vi "Revision Query.vi"(8 "error in (no error)":errorcluster, 11 "VISA resource name":refnum<visa-resource-name>) -> (0 "error out":errorcluster, 1 "Instrument Firmware Revision":string, 2 "Instrument Driver Revision":string, 3 "VISA resource name out":refnum<visa-resource-name>)   [LabVIEW 2015, in "Newport ESP301.lvlib"]
doc: "This command is used to read the controller type and version.\n\n<B>NOTE:</B> Important information needed when asking for technical support for the motion control system or when reporting a problem is the controller version. Use this command to determine the controller type and in particular, the firmware version.\n\nRefer to the Readme file for detailed driver information including modification history."
uses:
  <userlib>/Newport ESP301/Newport ESP301.lvlib
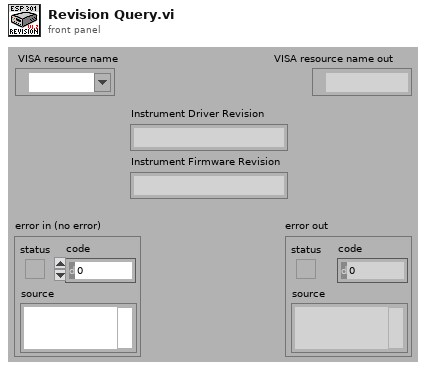
[diagram p1: front panel]
types:
  T1 = cluster{"Major":u16, "Minor":u16, "Fix":u16, "Build":u16}
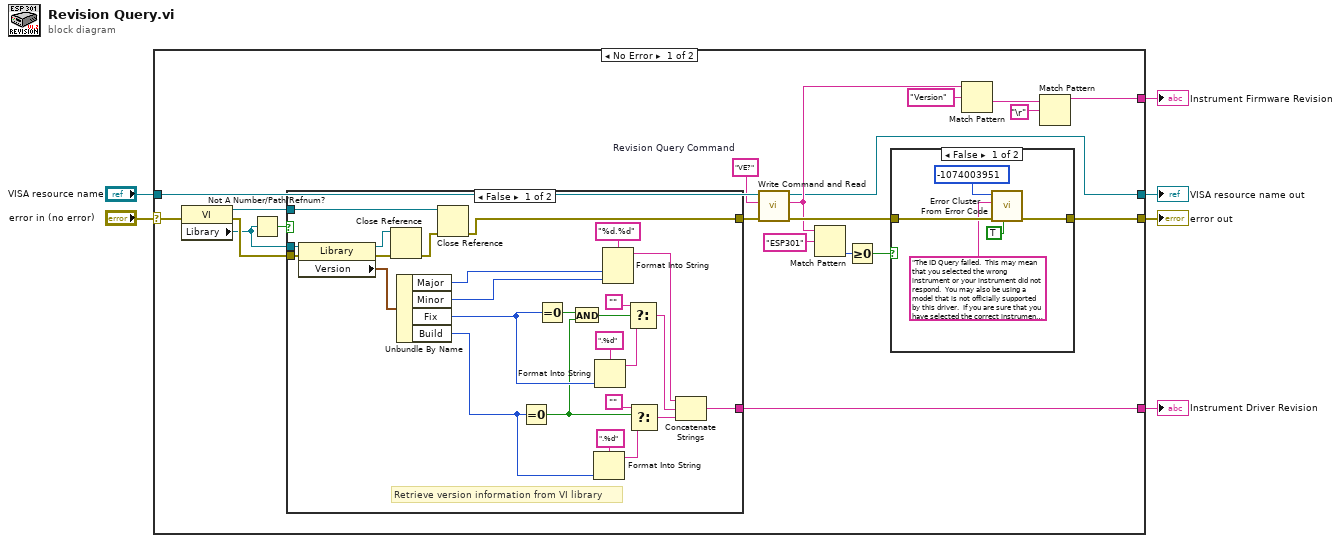
[diagram p0: block diagram]
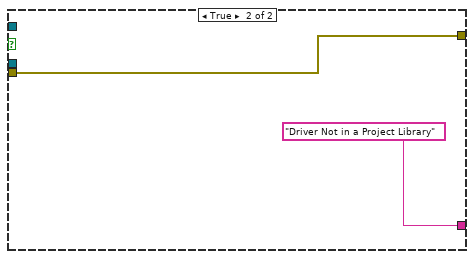
[diagram p3: hidden frame]
diagram:
  n1 = case shown="No Error" "error in (no error)" {
    selector: "error in (no error)" -> [w14 w62]
    tunnel: [w7 w61] -> w6
    tunnel: [w8 w62] -> w5
    tunnel: [w22 _] -> w4
    tunnel: [w18 _] -> w3
    tunnel: "VISA resource name" -> [w16 w61]
    frame No Error {
      w15 = "VE?"  # Revision Query Command
      n2 = property class="VI"(error in=w14) -> (reference out=w26:refnum<vi>, error out=w25:errorcluster, "Library"=w24:refnum<vi>)  [unwired: 1 in]
      n3 = Not A Number/Path/Refnum?(number/path/refnum=w24) -> (NaN/Path/Refnum?=w23:bool)
      n4 = case shown="False" w23 {
        tunnel: w26 -> [w55 _]
        tunnel: w25 -> [w40 w60]
        tunnel: [w35 w60] -> w17
        tunnel: [w34 "Driver Not in a Project Library"] -> w22
        tunnel: w24 -> [w33 _]
        frame False {
          # "Retrieve version information from VI library"
          n5 = property class="Library"(reference=w33, error in=w40) -> (reference out=w57:refnum<vi>, error out=w58:errorcluster, "Version"=w54:T1)
          n6 = Close Reference(reference=w57, error in (no error)=w58) -> (error out=w56:errorcluster)
          n7 = Unbundle By Name(w54) -> ("Major"=w43:u16, "Minor"=w42:u16, "Fix"=w39:u16, "Build"=w41:u16)
          n8 = Close Reference(reference=w55, error in (no error)=w56) -> (error out=w35:errorcluster)
          n9 = Equal To 0?(x=w41) -> (x = 0?=w37:bool)
          n10 = Equal To 0?(x=w39) -> (x = 0?=w38:bool)
          n11 = And(x=w38, y=w37) -> (x .and. y?=w36:bool)
          n12 = Format Into String(format string=".%d", w41) -> (resulting string=w47:string)  [unwired: 2 in, 1 out]
          n13 = Format Into String(format string=".%d", w39) -> (resulting string=w51:string)  [unwired: 2 in, 1 out]
          n14 = Format Into String(format string="%d.%d", w43, w42) -> (resulting string=w49:string)  [unwired: 2 in, 1 out]
          n15 = Select(t="", s=w36, f=w51) -> (s? t:f=w48:string)
          n16 = Select(t="", s=w37, f=w47) -> (s? t:f=w44:string)
          n17 = Concatenate Strings(w49, w48, w44) -> (w34:string)
        }
        frame True {
        }
      }
      n18 = call <userlib>:"Write Command and Read.vi"("error in (no error)"=w17, "Command"=w15, "VISA resource name"=w16) -> ("error out"=w13:errorcluster, "Returned string"=w12:string, "VISA resource name out"=w7:refnum<visa-resource-name>)  [unwired: 4 in]
      n19 = Match Pattern(string=w12, regular expression="ESP301") -> (offset past match=w10:i32)  [unwired: 1 in, 3 out]
      n20 = Greater Or Equal To 0?(x=w10) -> (x >= 0?=w9:bool)
      n21 = case shown="False" w9 {
        tunnel: w13 -> [w31 w32]
        tunnel: [w30 w32] -> w8
        frame False {
          n22 = call <vilib>:"Error Cluster From Error Code.vi"("show call chain? (False)"=TRUE, "error in (no error)"=w31, "error message (\"\")"="The ID Query failed.  This may mean that you selected the wrong instrument or your instrument did not respond.  You may also be using a model that is not officially supported by this driver.  If you are sure that you have selected the correct instrument and it is responding, try disabling the ID Query." ("Source (VI Name)"), "error code (0)"=-1074003951 ("Code")) -> ("error out"=w30:errorcluster)  [unwired: 5 in]
        }
        frame True {
        }
      }
      n23 = Match Pattern(string=w12, regular expression="Version" ("expression régulière")) -> (after substring=w20:string)  [unwired: 1 in, 3 out]
      n24 = Match Pattern(string=w20, regular expression="\r") -> (before substring=w18:string)  [unwired: 1 in, 3 out]
    }
    frame Error {
    }
  }
  "Instrument Firmware Revision" <- w3
  "Instrument Driver Revision" <- w4
  "VISA resource name out" <- w6
  "error out" <- w5
